vi "test type.vi"() -> ()   [LabVIEW 2020]
uses:
  9b7bf359-1e3f-4ca3-8efc-68bf7bf3cf6b.vi
  Nominal Client.lvclass
  f36276fe-c188-4252-be69-0cd9933e6484.vi
  type/type.lvclass
panel:
  out "createdAt":timestamp
  in  "name 2":string
  out "name":string
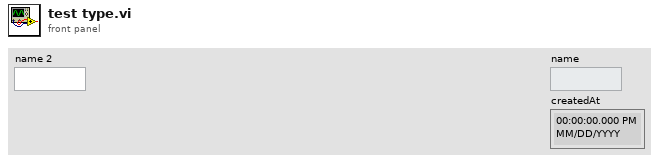
[diagram p1: front panel]
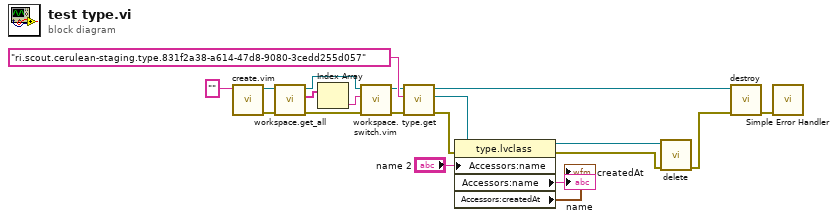
[diagram p0: block diagram]
diagram:
  n1 = call "create.vim"("API Token (string or path)"="") -> ("error out"=w13:errorcluster, "Nominal Client"=w14:refnum<class "Nominal Client.lvclass">)  [unwired: 9 in]
  n2 = call "workspace.get_all.vi"("error in"=w13, "Nominal Client in"=w14) -> ("error out"=w16:errorcluster, "Workspace RIDs"=w17:string[], "Nominal Client out"=w18:refnum<class "Nominal Client.lvclass">)  [unwired: 5 in, 2 out]
  n3 = Index Array(array=w17) -> (element=w15:string)  [unwired: 1 in]
  n4 = call "workspace.switch.vim"("error in"=w16, "Workspace RID (string or path)"=w15, "Nominal Client in"=w18) -> ("error out"=w10:errorcluster, "Nominal Client out"=w11:refnum<class "Nominal Client.lvclass">)  [unwired: 7 in]
  n5 = call "type.get.vi"("error in"=w10, "Type RID"="ri.scout.cerulean-staging.type.831f2a38-a614-47d8-9080-3cedd255d057" ("API Token (string or path)"), "Nominal Client in"=w11) -> ("error out"=w5:errorcluster, "type"=w8:refnum<class "type.lvclass">, "Nominal Client out"=w9:refnum<class "Nominal Client.lvclass">)  [unwired: 6 in]
  n6 = property class="type.lvclass"(reference=w8, error in=w5, "Accessors:name"="name 2") -> (reference out=w3:refnum<class "type.lvclass">, error out=w2:errorcluster, "Accessors:name"=→"name":string, "Accessors:createdAt"=→"createdAt":timestamp)
  n7 = call "delete.vi"("error in"=w2, "type in"=w3) -> ("error out"=w1:errorcluster)  [unwired: 8 in, 1 out]
  n8 = call "destroy.vi"("error in"=w1, "Nominal Client"=w9) -> ("error out"=w19:errorcluster)  [unwired: 9 in]
  n9 = call <vilib>:"Simple Error Handler.vi"("error in (no error)"=w19) -> ()  [unwired: 4 in, 5 out]
